vi "Set TCP Messaging.vi"(8 "error in (no error)":errorcluster, 10 "Messaging":refnum<class "TCPMessageAPI.lvclass">, 11 "VolatusAPI in":refnum<class "VolatusAPI.lvclass">) -> (0 "error out":errorcluster, 3 "VolatusAPI out":refnum<class "VolatusAPI.lvclass">)   [LabVIEW 2020, in "Volatus.lvlib" / "VolatusAPI.lvclass"]
uses:
  VolatusAPI.lvclass
  VolatusAPI.lvclass/VolatusAPI.ctl
  lv-vecto/Vecto/TCPMessageService/TCPMessageAPI.lvclass
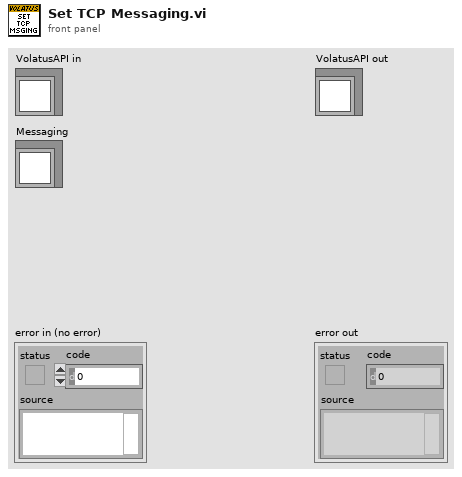
[diagram p1: front panel]
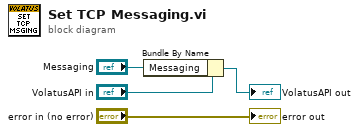
[diagram p0: block diagram]
diagram:
  n1 = Bundle By Name(cluster="VolatusAPI in", "Messaging"="Messaging") -> (→"VolatusAPI out":refnum<class "VolatusAPI.lvclass">)
  "error out" <- "error in (no error)"
